vi "Head Filter Tests.vi"() -> ()   [LabVIEW 2017]
uses:
  <vilib>/Analysis/3filter.llb/Filter Passband Type.ctl
  <vilib>/ptbypt/NI_PtbyPt.lvlib
  <vilib>/Analysis/NI_AALBase.lvlib
panel:
  out "Filtered":dbl[](graph)
  out "Raw":dbl[](graph)
  in  "low cutoff freq: fl":dbl=0.125 format="%0.3f"
  out "Oculus Data":T1
  out "error out":errorcluster
  out "String":string
  in  "stop":bool
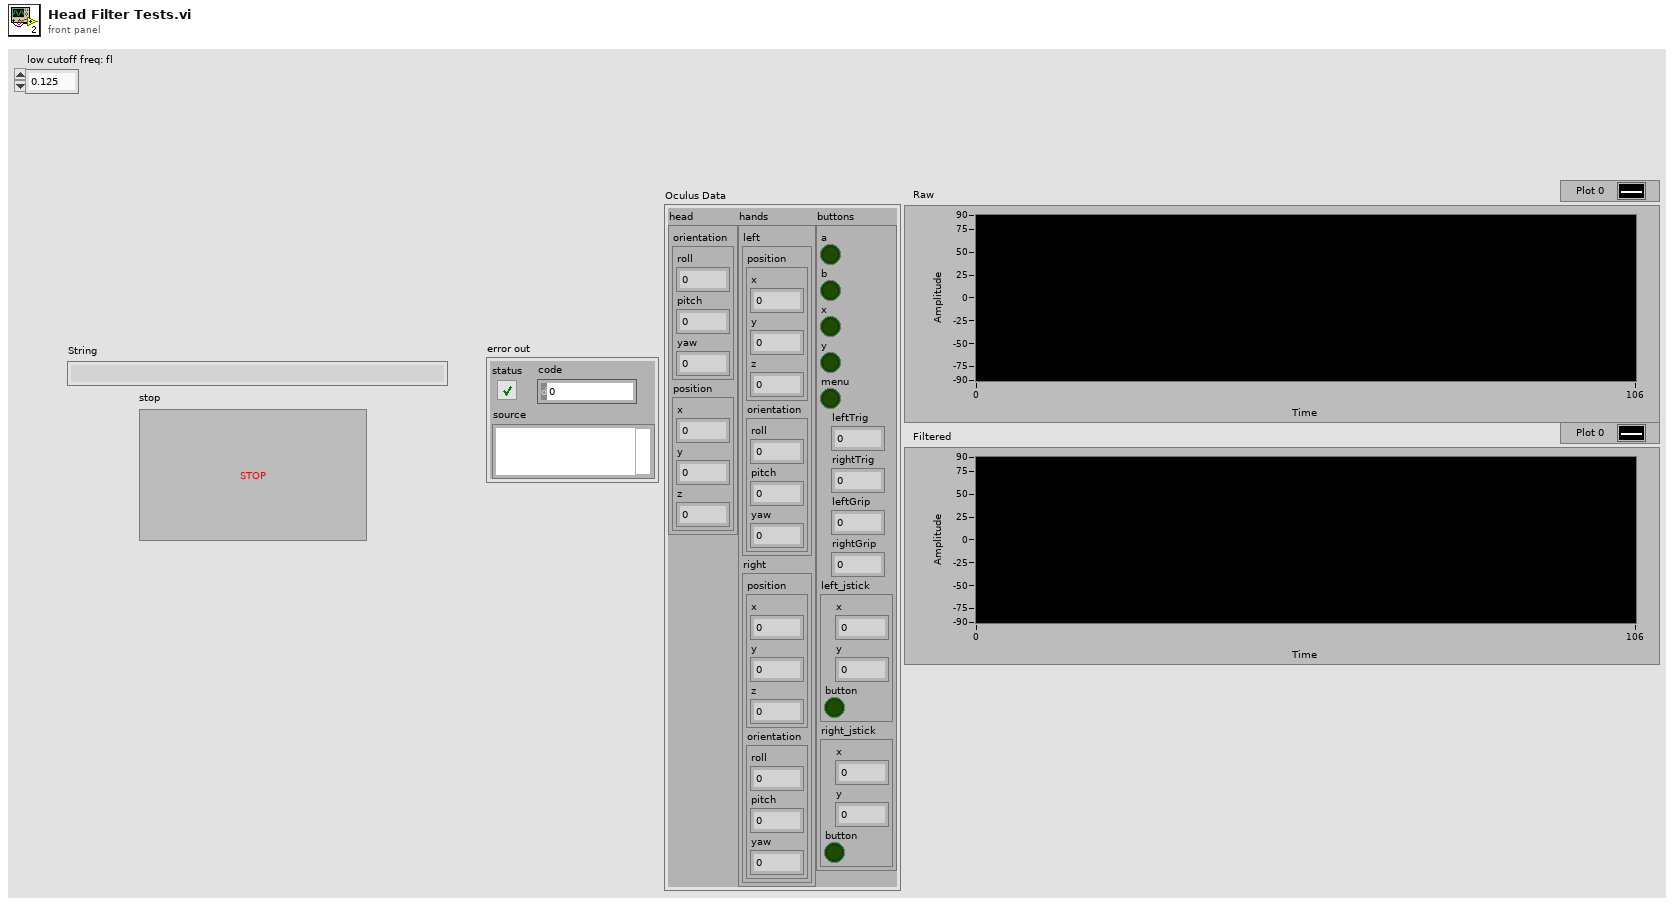
[diagram p1: front panel]
types:
  T1 = cluster{"head":cluster{"orientation":cluster{"roll":dbl, "pitch":dbl, "yaw":dbl}, "position":cluster{"x":dbl, "y":dbl, "z":dbl}}, "hands":cluster{"left":cluster{"position":cluster{"x":dbl, "y":dbl, "z":dbl}, "orientation":cluster{"roll":dbl, "pitch":dbl, "yaw":dbl}}, "right":cluster{"position":cluster{"x":dbl, "y":dbl, "z":dbl}, "orientation":cluster{"roll":dbl, "pitch":dbl, "yaw":dbl}}}, "buttons":cluster{"a":bool, "b":bool, "x":bool, "y":bool, "menu":bool, "leftTrig":dbl, "rightTrig":dbl, "leftGrip":dbl, "rightGrip":dbl, "left_jstick":cluster{"x":dbl, "y":dbl, "button":bool}, "right_jstick":cluster{"x":dbl, "y":dbl, "button":bool}}}
  T2 = typedef "NI_AALBase.lvlib/Filter Passband Type.ctl" = enum32{"Lowpass", "Highpass", "Bandpass", "Bandstop"}
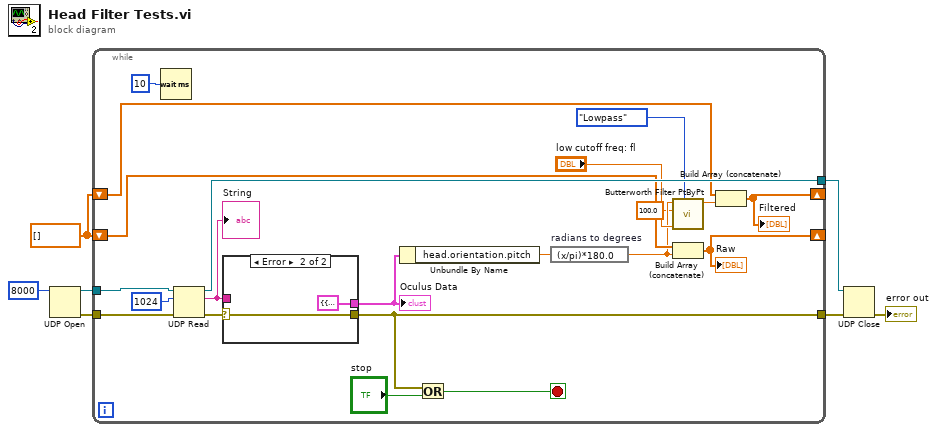
[diagram p0: block diagram]
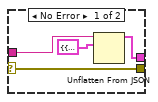
[diagram p2: hidden frame]
diagram:
  w1 = dbl[] []
  n1 = UDP Open(11:8000) -> (port=w5:refnum<k16>, 0:w6:errorcluster)  [unwired: 4 in, 1 out]
  n2 = while {
    tunnel: w6 -> [w28]
    tunnel: w5 -> [w27]
    tunnel: [w26] -> w4
    tunnel: [w20] -> w2
    shift-right: [w11] -> _
    shift-left: w1 -> [w15]
    shift-right: [w12] -> _
    shift-left: w1 -> [w13]
    stop <- w19 stop-if-true
    n3 = Wait (ms)(milliseconds to wait=u32 10) -> ()  [unwired: 1 out]
    n4 = UDP Read(connection ID=w27, max size (548)=1024, 8:w28) -> (data out=w23:string, error out=w24:errorcluster, 3:w26:refnum<k16>)  [unwired: 1 in, 2 out]
    "String" <- w23
    n5 = case shown="Error" w24 {
      selector: w24 -> [w31 w34]
      tunnel: [w31 w34] -> w20
      tunnel: w23 -> [w32 _]
      tunnel: [w30 T1 {"head"={"orientation"={"roll"=3.1657064096568246, "pitch"=-11.484824411838325, "yaw"=9.16228269349602}, "position"={"x"=0.695052, "y"=0.072933, "z"=-0.662641}}, "hands"={"left"={"position"={"x"=316.12422992289123, "y"=-278.4992818124042, "z"=55.442337434288575}, "orientation"={"roll"=11.516910048365652, "pitch"=-12.32140008850884, "yaw"=25.887952057395985}}, "right"={"position"={"x"=258.10388614691647, "y"=-336.1085821074321, "z"=-158.28405769322922}, "orientation"={"roll"=9.049925669870866, "pitch"=-89.22253484381864, "yaw"=-45.57672995459452}}}, "buttons"={"a"=FALSE, "b"=FALSE, "x"=FALSE, "y"=FALSE, "menu"=TRUE, "leftTrig"=1e-06, "rightTrig"=1e-06, "leftGrip"=0.995147, "rightGrip"=1e-06, "left_jstick"={"x"=0.0, "y"=0.0, "button"=FALSE}, "right_jstick"={"x"=0.0, "y"=0.0, "button"=FALSE}}} ("Oculus Data in")] -> w18
      frame No Error {
        n6 = Unflatten From JSON(JSON string=w32, type and defaults=T1 {"head"={"orientation"={"roll"=3.1657064096568246, "pitch"=-11.484824411838325, "yaw"=9.16228269349602}, "position"={"x"=0.695052, "y"=0.072933, "z"=-0.662641}}, "hands"={"left"={"position"={"x"=316.12422992289123, "y"=-278.4992818124042, "z"=55.442337434288575}, "orientation"={"roll"=11.516910048365652, "pitch"=-12.32140008850884, "yaw"=25.887952057395985}}, "right"={"position"={"x"=258.10388614691647, "y"=-336.1085821074321, "z"=-158.28405769322922}, "orientation"={"roll"=9.049925669870866, "pitch"=-89.22253484381864, "yaw"=-45.57672995459452}}}, "buttons"={"a"=FALSE, "b"=FALSE, "x"=FALSE, "y"=FALSE, "menu"=TRUE, "leftTrig"=1e-06, "rightTrig"=1e-06, "leftGrip"=0.995147, "rightGrip"=1e-06, "left_jstick"={"x"=0.0, "y"=0.0, "button"=FALSE}, "right_jstick"={"x"=0.0, "y"=0.0, "button"=FALSE}}} ("Oculus Data in")) -> (value=w30:T1)  [unwired: 5 in, 1 out]
      }
      frame Error {
      }
    }
    "Oculus Data" <- w18
    n7 = Unbundle By Name(w18) -> ("head.orientation.pitch"=w10:dbl)
    n8 = Or(x=w20, y="stop") -> (x .or. y?=w19:bool)
    n9 = expression code="(x/pi)*180.0" "radians to degrees"(w10) -> (w9:dbl)
    n10 = call <vilib>:"Butterworth Filter PtByPt.vi"("filter type"=Filter_Passband_Type."Lowpass", "low cutoff freq: fl"="low cutoff freq: fl", "sampling freq: fs"=100.0, "x"=w9) -> ("Filtered x"=w14:dbl)  [unwired: 5 in, 1 out]
    n11 = Build Array (concatenate)(w13, w9) -> (w12:dbl[])
    "Raw" <- w12
    n12 = Build Array (concatenate)(w15, w14) -> (w11:dbl[])
    "Filtered" <- w11
  }
  n13 = UDP Close(connection ID=w4, 8:w2) -> (error out=→"error out":errorcluster)  [unwired: 1 out]
